vi "Find Control in Cluster.vi"(8 "error in (no error)":errorcluster, 10 "String":string, 11 "Controls[]":refnum<vi>[](array[refnum])) -> (0 "error out":errorcluster, 3 "Control out":refnum<vi>)   [LabVIEW 2014]
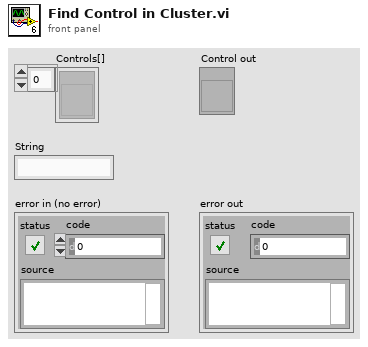
[diagram p1: front panel]
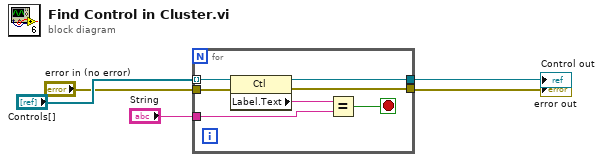
[diagram p0: block diagram]
diagram:
  n1 = for {
    tunnel: "Controls[]" -> [w12] mode=indexing
    tunnel: "error in (no error)" -> [w11]
    tunnel: "String" -> [w9]
    tunnel: [w8] -> w4
    tunnel: [w6] -> w5
    stop <- w7 stop-if-true
    n2 = property class="Ctl"(reference=w12, error in=w11) -> (reference out=w6:refnum<vi>, error out=w8:errorcluster, "Label.Text"=w10:string)
    n3 = Equal?(x=w10, y=w9) -> (x = y?=w7:bool)
  }
  "Control out" <- w5
  "error out" <- w4
